vi "Change Table Cell Size.vi"(10 "Column":u32, 11 "RobotPoint":refnum<vi>) -> ()   [LabVIEW 2019]
uses:
  <vilib>/Utility/miscctls.llb/LVRowAndColumnUnsignedTypeDef.ctl
  <vilib>/Utility/miscctls.llb/LVBoundsTypeDef.ctl
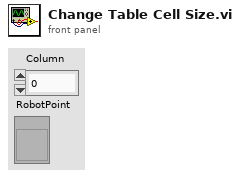
[diagram p1: front panel]
types:
  T1 = typedef "LVBoundsTypeDef.ctl" = cluster{"Width":u32, "Height":u32}
  T2 = typedef "LVRowAndColumnUnsignedTypeDef.ctl" = cluster{"Row":u32, "Column":u32}
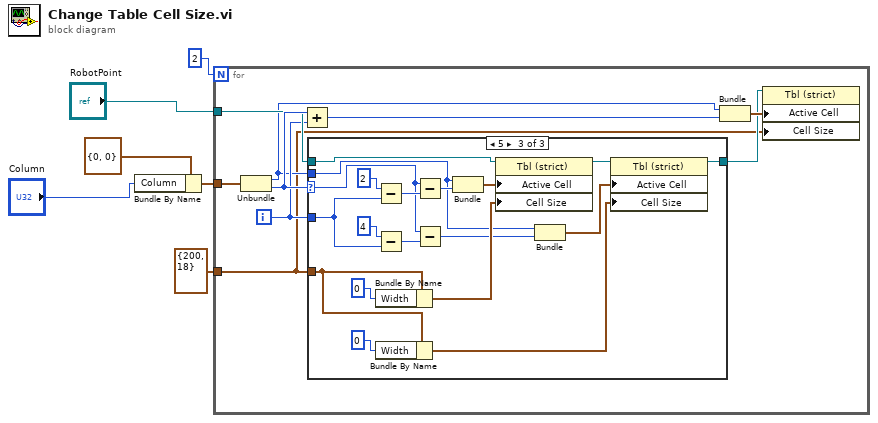
[diagram p0: block diagram]
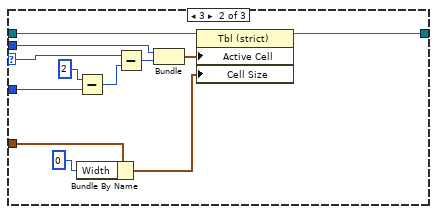
[diagram p3: hidden frame]
diagram:
  n1 = Bundle By Name(cluster=T2 {"Row"=0, "Column"=0} ("Index Values"), "Column"="Column") -> (w3:T2)
  n2 = for {
    N: 2 -> [_]
    tunnel: w3 -> [w15]
    tunnel: "RobotPoint" -> [w11]
    tunnel: T1 {"Width"=200, "Height"=18} ("Active Cell:Cell Size") -> [w7]
    i -> [w9]
    n3 = Unbundle(w15) -> ("Row"=w8:u32, "Column"=w12:u32)
    n4 = Add(x=w12, y=w9) -> (x+y=w14:u32)
    n5 = case shown="5" w12 {
      selector: w12 -> [_ w26 w30]
      tunnel: w11 -> [w16 w28 w47]
      tunnel: [w16 w27 w34] -> w10
      tunnel: w9 -> [_ w17 w29]
      tunnel: w8 -> [_ w23 w32]
      tunnel: w7 -> [_ w21 w31]
      frame 0, Default {
      }
      frame 3 {
        n6 = Subtract(x=2 ("y"), y=w17) -> (x-y=w25:i32)
        n7 = Bundle By Name(cluster=w21, "Width"=u32 0) -> (w19:T1)
        n8 = Subtract(x=w26, y=w25) -> (x-y=w24:u32)
        n9 = Bundle("Row"=w23, w24) -> (w22:cluster{"Row":u32, u32})  [unwired: 1 in]
        n10 = property on="Property Node" class="Tbl (strict)"(reference=w28, "Active Cell"=w22, "Cell Size"=w19) -> (reference out=w27:refnum<vi>)  [unwired: 1 in, 1 out]
      }
      frame 5 {
        n11 = Subtract(x=2 ("y"), y=w29) -> (x-y=w46:i32)
        n12 = Subtract(x=4 ("y"), y=w29) -> (x-y=w35:i32)
        n13 = Bundle By Name(cluster=w31, "Width"=u32 0) -> (w41:T1)
        n14 = Bundle By Name(cluster=w31, "Width"=u32 0) -> (w40:T1)
        n15 = Subtract(x=w30, y=w46) -> (x-y=w44:u32)
        n16 = Subtract(x=w30, y=w35) -> (x-y=w37:u32)
        n17 = Bundle("Row"=w32, w44) -> (w43:cluster{"Row":u32, u32})  [unwired: 1 in]
        n18 = property on="Property Node" class="Tbl (strict)"(reference=w47, "Active Cell"=w43, "Cell Size"=w41) -> (reference out=w33:refnum<vi>)  [unwired: 1 in, 1 out]
        n19 = Bundle("Row"=w32, w37) -> (w38:cluster{"Row":u32, u32})  [unwired: 1 in]
        n20 = property on="Property Node" class="Tbl (strict)"(reference=w33, "Active Cell"=w38, "Cell Size"=w40) -> (reference out=w34:refnum<vi>)  [unwired: 1 in, 1 out]
      }
    }
    n21 = Bundle("Row"=w8, w14) -> (w13:cluster{"Row":u32, u32})  [unwired: 1 in]
    n22 = property on="Property Node" class="Tbl (strict)"(reference=w10, "Active Cell"=w13, "Cell Size"=w7) -> ()  [unwired: 1 in, 2 out]
  }
